vi "KB To MB.vi"(11 "KB":dbl) -> (3 "MB":dbl)   [LabVIEW 2020, in "RTAF.lvlib" / "System Status Actor.lvclass"]
uses:
  System Status Actor.lvclass
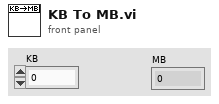
[diagram p1: front panel]
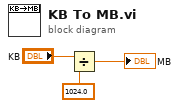
[diagram p0: block diagram]
diagram:
  n1 = Divide(x="KB", y=1024.0) -> (x/y=→"MB":dbl)
